vi "Create WFG Plug In List.vi"(0 "path":path) -> (2 "menu names":string[](array[string]), 3 "VI paths":path[](array[path]), 4 "Error":errorcluster[](array[cluster]))   [LabVIEW 2011]
doc: "Reads the plugins directory. Any VIs which are contained in the directory are opened according to the type specifier on the front panel of this VI. If the vi is successfully opened the Title of the VIs window is read and placed in a list which will be used to create a selection list.\n\nAAL 9/09"
panel:
  in  "type specifier VI refnum":refnum<vi>
  # "Reads the plugins directory.  Any VIs which are contained in the directory \nare opened according to the type specifier on the front panel of this VI.  \nIf the vi is successfully opened the Title of the VIs window is read and placed \nin a list which will be used to create a selection list."
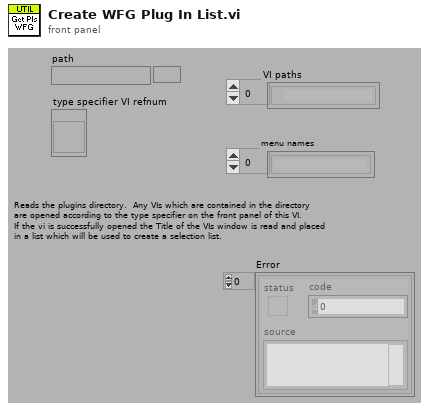
[diagram p1: front panel]
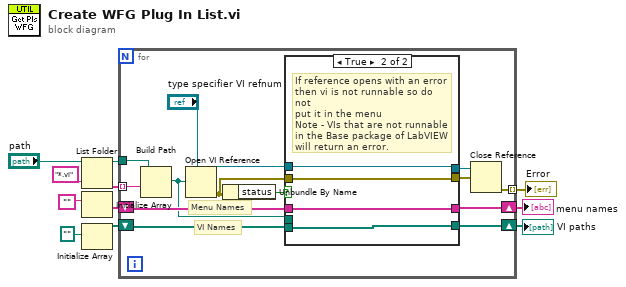
[diagram p0: block diagram]
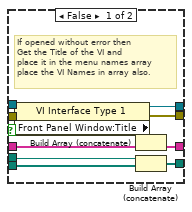
[diagram p2: hidden frame]
diagram:
  n1 = List Folder(path="path", pattern="*.vi") -> (path out=w3:path, filenames=w11:string[])  [unwired: 1 in, 3 out]
  n2 = Initialize Array("") -> (w6:string[])  [unwired: 1 out]
  n3 = Initialize Array(path "") -> (w4:path[])  [unwired: 1 out]
  n4 = for {
    tunnel: w11 -> [w15] mode=indexing
    tunnel: w3 -> [w25]
    shift-right: [w21] -> w7
    shift-left: w6 -> [w22]
    shift-right: [w13] -> w8
    shift-left: w4 -> [w18]
    tunnel: [w12] -> w1 mode=indexing
    # "Menu Names"
    # "VI Names"
    n5 = Build Path(base path=w25, name or relative path=w15) -> (appended path=w14:path)
    n6 = Open VI Reference(type specifier VI Refnum (for type only)="type specifier VI refnum", vi path=w14) -> (vi reference=w20:refnum<vi>, error out=w19:errorcluster)  [unwired: 2 in, 2 out]
    n7 = Unbundle By Name(w19) -> ("status"=w23:bool)
    n8 = case shown="True" w23 {
      tunnel: w22 -> [w32 w39]
      tunnel: [w31 w39] -> w21
      tunnel: w20 -> [w35 w37]
      tunnel: w19 -> [w34 w38]
      tunnel: w18 -> [w27 w36]
      tunnel: [w30 w36] -> w13
      tunnel: w14 -> [w26 _]
      tunnel: [w29 w37] -> w17
      tunnel: [w28 w38] -> w16
      frame False {
        # "If opened without error then\nGet the Title of the VI and \nplace it in the menu names array\nplace the VI Names in array also."
        n9 = property class="VI Interface Type 1"(reference=w35, error in=w34) -> (reference out=w29:refnum<vi>, error out=w28:errorcluster, "Front Panel Window:Title"=w33:string)
        n10 = Build Array (concatenate)(w33, w32) -> (w31:string[])
        n11 = Build Array (concatenate)(w26, w27) -> (w30:path[])
      }
      frame True {
        # "If reference opens with an error\nthen vi is not runnable so do not\nput it in the menu\nNote - VIs that are not runnable\nin the Base package of LabVIEW\nwill return an error."
      }
    }
    n12 = Close Reference(reference=w17, error in (no error)=w16) -> (error out=w12:errorcluster)
  }
  "VI paths" <- w8
  "menu names" <- w7
  "Error" <- w1
